vi "Discharge Main.vi"() -> ()   [LabVIEW 2012]
uses:
  Generic Instrument/Data Logger/Data Logger.lvclass
panel:
  out "New set":dbl
  out "Absolute Current set":dbl
  out "Cut-Off Voltage":dbl
  out "Calculated DOD":dbl
  out "Voltage cut off?":bool
  out "Amp hour?":bool
  out "Chroma Load":errorcluster caption="error out" {"code" format="%.0x"}
  out "WT1600":errorcluster
  out "Amp-Hour":dbl
  out "Watt-Hour":dbl
  out "Power":dbl
  out "Current":dbl
  out "Measure":dbl[](array[numeric]) format="%^.4e"
  out "Voltage":dbl
  in  "WT1600":refnum<visa-resource-name>="GPIB0::10::INSTR"
  in  "Chroma 6320 Load":refnum<k15>="GPIB::5::INSTR" caption="resource name"
  out "Time":dbl format="%<%H:%M:%S>t"
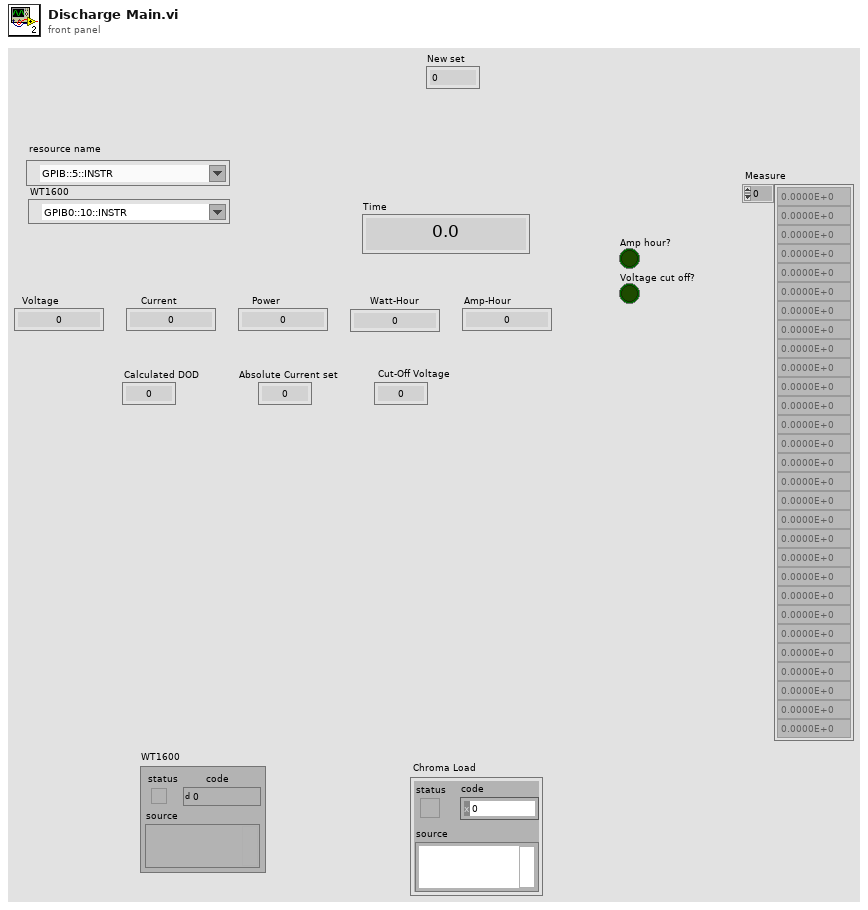
[diagram p1: front panel]
types:
  T1 = cluster{"Amp-Hours":dbl, "% Depth Of Discharge":dbl, "Cut-Off Voltage":dbl}
  T2 = cluster{"Project":string, "Manufactuere":string, "Model":string, "Notes":string}
  T3 = cluster{"V Range (12: 1000)":u16, "A Range (9: 5A)":u16, "A Sensor Ratio(mV/A) (10.0000) ":dbl, "Wiring A (0: 1P2W)":u16}
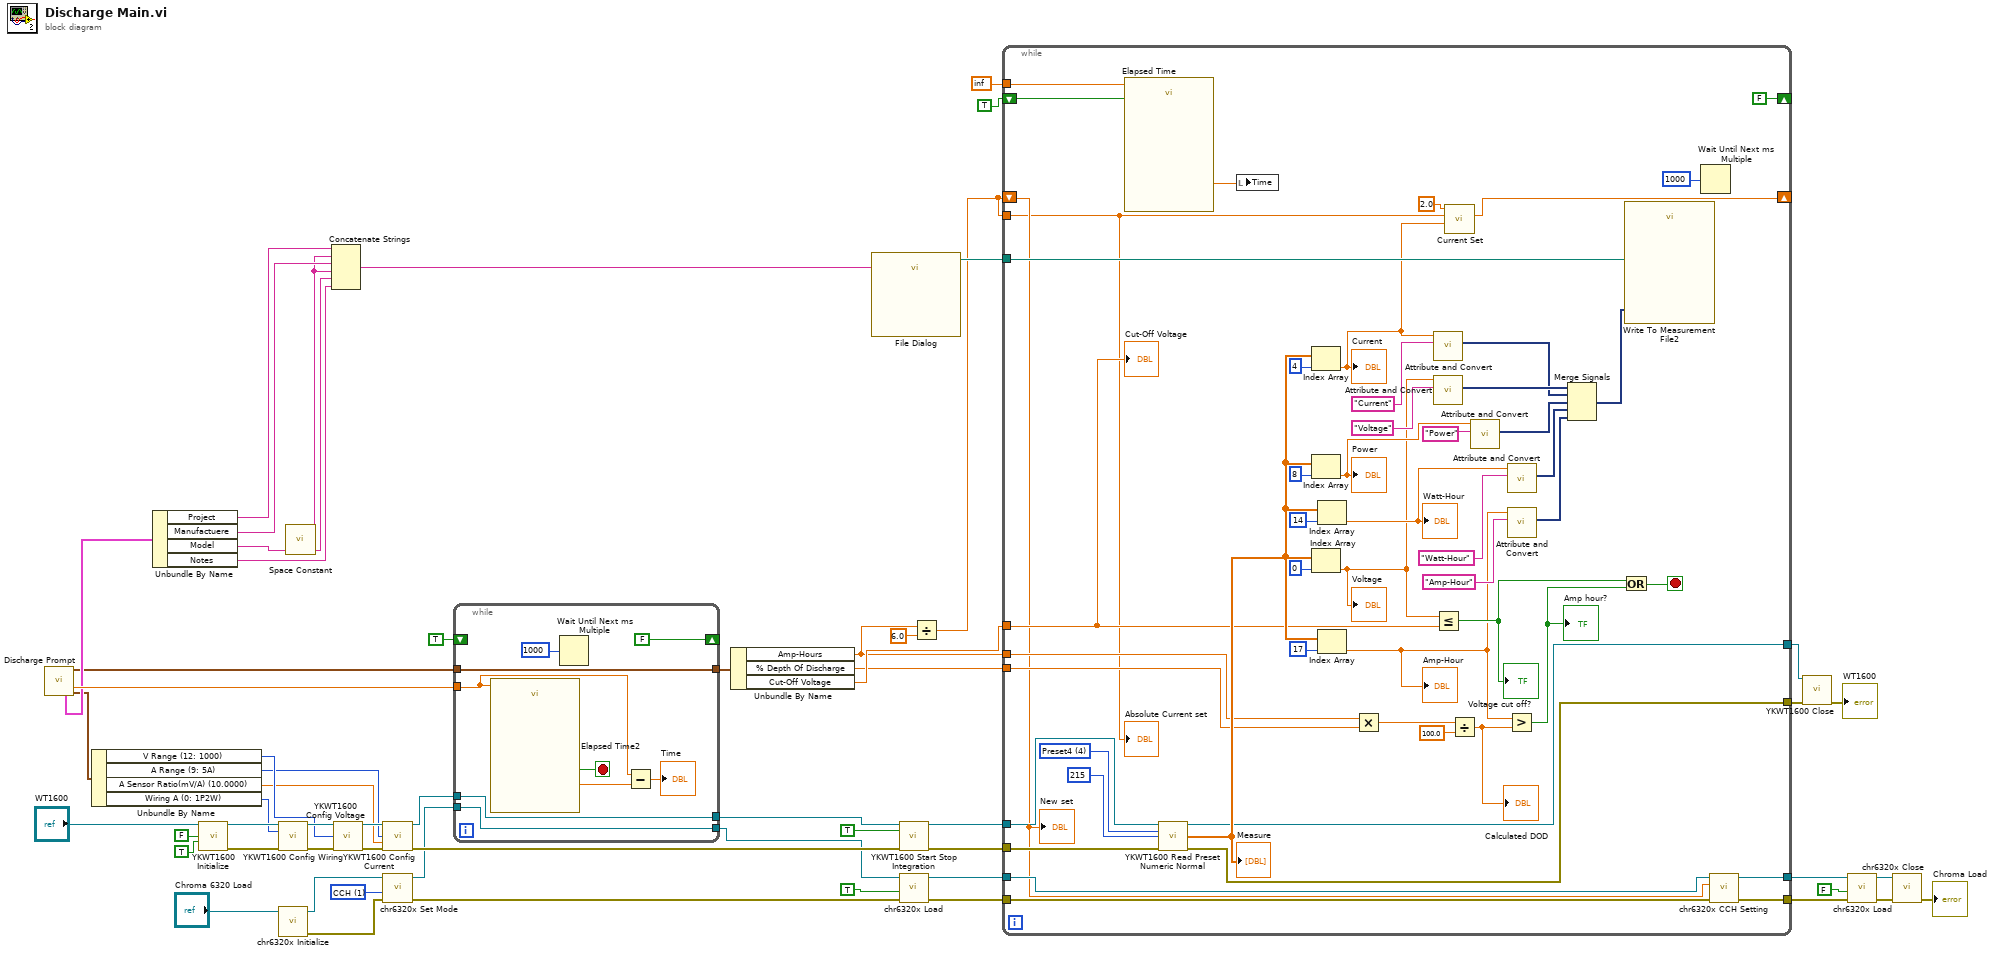
[diagram p0: block diagram]
diagram:
  w53 = 1 items=["CCL", "CCH", "CCDL", "CCDH", "CRL", "CRH", "CVL", "CVH", "CPL", "CPH", "CCEL", "CCEH"] ("Mode (CCL)")
  n1 = call "Discharge Prompt.vi"() -> ("output cluster"=w43:T1, "Warm-Up"=w58:dbl, "Cluster"=w52:T2, "Cluster 2"=w36:T3)  [unwired: 12 in]
  n2 = Unbundle By Name(w36) -> ("V Range (12: 1000)"=w34:u16, "A Range (9: 5A)"=w31:u16, "A Sensor Ratio(mV/A) (10.0000)"=w30:dbl, "Wiring A (0: 1P2W)"=w35:u16)
  n3 = Unbundle By Name(w52) -> ("Project"=w51:string, "Manufactuere"=w50:string, "Model"=w49:string, "Notes"=w47:string)
  n4 = call <instrlib>:"YKWT1600 Initialize.vi"("VISA session (for class)"="WT1600", "ID Query (T: Check)"=FALSE, "Reset (T: Reset)"=TRUE) -> ("VISA session"=w40:refnum<visa-resource-name>, "error out"=w39:errorcluster)  [unwired: 11 in]
  n5 = call <instrlib>:"YKWT1600 Config Wiring.vi"("VISA session"=w40, "Wiring A (0: 1P2W)"=w35, "error in (no error)"=w39) -> ("dup VISA session"=w38:refnum<visa-resource-name>, "error out"=w37:errorcluster)  [unwired: 11 in]
  n6 = call <instrlib>:"chr6320x Initialize.vi"("resource name"="Chroma 6320 Load") -> ("error out"=w54:errorcluster, "instrument handle out"=w55:refnum<k15>)  [unwired: 9 in]
  n7 = call <vilib>:"Space Constant.vi"() -> ("String"=w48:string)
  n8 = Concatenate Strings(w51, w48, w50, w48, w49, w47) -> (w46:string)
  n9 = call <instrlib>:"YKWT1600 Config Voltage.vi"("VISA session"=w38, "V Range (12: 1000)"=w34, "error in (no error)"=w37) -> ("dup VISA session"=w33:refnum<visa-resource-name>, "error out"=w32:errorcluster)  [unwired: 11 in]
  n10 = call <instrlib>:"YKWT1600 Config Current.vi"("VISA session"=w33, "A Range (9: 5A)"=w31, "A Sensor Ratio(mV/A) (10.0000)"=w30, "error in (no error)"=w32) -> ("dup VISA session"=w29:refnum<visa-resource-name>, "error out"=w26:errorcluster)  [unwired: 10 in]
  n11 = call <instrlib>:"chr6320x Set Mode.vi"("error in (no error)"=w54, "Mode (CCL)"=w53, "instrument handle"=w55) -> ("error out"=w19:errorcluster, "instrument handle out"=w20:refnum<k15>)  [unwired: 7 in]
  n12 = while {
    tunnel: w58 -> [w64]
    shift-right: [FALSE] -> _
    shift-left: TRUE -> [_]
    tunnel: [w61] -> w22
    tunnel: w43 -> [w61]
    tunnel: [w60] -> w28
    tunnel: w29 -> [w60]
    tunnel: [w59] -> w17
    tunnel: w20 -> [w59]
    stop <- w66 stop-if-true
    n13 = call "Elapsed Time2"("Time Target (s)"=w64) -> ("Elapsed Time (s)"=w63:dbl, "Time has Elapsed"=w66:bool)  [unwired: 11 in, 6 out]
    n14 = Wait Until Next ms Multiple(millisecond multiple=u32 1000) -> ()  [unwired: 1 out]
    n15 = Subtract(x=w64, y=w63) -> (x-y=→"Time":dbl)
  }
  n16 = Unbundle By Name(w22) -> ("Amp-Hours"=w3:dbl, "% Depth Of Discharge"=w4:dbl, "Cut-Off Voltage"=w21:dbl)
  n17 = call "File Dialog"("default name"=w46) -> ("selected path"=w5:path)  [unwired: 11 in, 3 out]
  n18 = call <instrlib>:"YKWT1600 Start Stop Integration.vi"("VISA session"=w28, "Start/Stop (F: Stop)"=TRUE, "error in (no error)"=w26) -> ("dup VISA session"=w27:refnum<visa-resource-name>, "error out"=w25:errorcluster)  [unwired: 11 in]
  n19 = call <instrlib>:"chr6320x Load.vi"("error in (no error)"=w19, "Load (On)"=TRUE, "instrument handle"=w17) -> ("error out"=w15:errorcluster, "instrument handle out"=w16:refnum<k15>)  [unwired: 7 in]
  n20 = Divide(x=w3, y=6.0) -> (x/y=w1:dbl)
  n21 = while {
    tunnel: w16 -> [w88]
    tunnel: w15 -> [w89]
    shift-right: [FALSE] -> _
    shift-left: TRUE -> [w117]
    tunnel: inf -> [w115]
    tunnel: w27 -> [w113]
    tunnel: w25 -> [w112]
    tunnel: w5 -> [w103]
    tunnel: w3 -> [w83]
    tunnel: w21 -> [w85]
    tunnel: w4 -> [w82]
    tunnel: [w79] -> w14
    tunnel: [w78] -> w13
    tunnel: [w77] -> w9
    tunnel: [w76] -> w8
    shift-right: [w71] -> _
    shift-left: w1 -> [w72]
    tunnel: w1 -> [w69]
    stop <- w87 stop-if-true
    w111 = u16 4 items=["", "Preset1", "Preset2", "Preset3", "Preset4"] ("Preset (2: Preset 2)")
    n22 = call "Elapsed Time"("Time Target (s)"=w115, "Reset"=w117) -> ("Elapsed Time (s)"=w114:dbl)  [unwired: 10 in, 7 out]
    n23 = call <instrlib>:"YKWT1600 Read Preset Numeric Normal.vi"("VISA session"=w113, "Preset (2: Preset 2)"=w111, "Number of Item (15)"=u16 215, "error in (no error)"=w112) -> ("dup VISA session"=w77:refnum<visa-resource-name>, "Measure"=w108:dbl[], "error out"=w76:errorcluster)  [unwired: 8 in, 1 out]
    "Measure" <- w108
    n24 = local write "Time"(w114) -> ()
    n25 = Index Array(array=w108, index=4) -> (element=w68:dbl)
    "Current" <- w68
    n26 = Index Array(array=w108, index=8) -> (element=w100:dbl)
    "Power" <- w100
    n27 = Index Array(array=w108, index=0) -> (element=w86:dbl)
    "Voltage" <- w86
    n28 = Index Array(array=w108, index=14) -> (element=w98:dbl)
    "Watt-Hour" <- w98
    n29 = Index Array(array=w108, index=17) -> (element=w81:dbl)
    "Amp-Hour" <- w81
    n30 = Multiply(x=w83, y=w82) -> (x*y=w75:dbl)
    n31 = call "Attribute and Convert.vi"("Signal Name"="Current", "Number in"=w68) -> ("Dynamic Signal Out"=w94:dynamicdata)  [unwired: 9 in]
    n32 = call "Attribute and Convert.vi"("Signal Name"="Voltage", "Number in"=w86) -> ("Dynamic Signal Out"=w95:dynamicdata)  [unwired: 9 in]
    n33 = Less Or Equal?(x=w86, y=w85) -> (x <= y?=w84:bool)
    "Voltage cut off?" <- w84
    n34 = call "Current Set.vi"("Actual Number"=w68, "Target"=w69, "Percent ceiling"=2.0) -> ("New Set Point"=w71:dbl)  [unwired: 8 in]
    n35 = Divide(x=w75, y=100.0) -> (x/y=w73:dbl)
    "Calculated DOD" <- w73
    n36 = call "Attribute and Convert.vi"("Signal Name"="Power", "Number in"=w100) -> ("Dynamic Signal Out"=w93:dynamicdata)  [unwired: 9 in]
    n37 = call "Attribute and Convert.vi"("Signal Name"="Watt-Hour", "Number in"=w98) -> ("Dynamic Signal Out"=w92:dynamicdata)  [unwired: 9 in]
    n38 = call "Attribute and Convert.vi"("Signal Name"="Amp-Hour", "Number in"=w81) -> ("Dynamic Signal Out"=w91:dynamicdata)  [unwired: 9 in]
    n39 = Greater?(x=w81, y=w73) -> (0:w80:bool)
    "Amp hour?" <- w80
    n40 = Merge Signals(w95, w94, w93, w92, w91) -> (w90:dynamicdata)
    n41 = Or(x=w84, y=w80) -> (x .or. y?=w87:bool)
    n42 = call "Write To Measurement File2"("Signals"=w90, "Filename"=w103) -> ()  [unwired: 15 in, 3 out]
    n43 = Wait Until Next ms Multiple(millisecond multiple=u32 1000) -> ()  [unwired: 1 out]
    n44 = call <instrlib>:"chr6320x CCH Setting.vi"("error in (no error)"=w89, "Current Level (0.0)"=w72, "instrument handle"=w88) -> ("error out"=w78:errorcluster, "instrument handle out"=w79:refnum<k15>)  [unwired: 7 in]
    "Cut-Off Voltage" <- w85
    "Absolute Current set" <- w69
    "New set" <- w72
  }
  n45 = call <instrlib>:"YKWT1600 Close.vi"("VISA session"=w9, "error in (no error)"=w8) -> ("error out"=→"WT1600":errorcluster)  [unwired: 13 in]
  n46 = call <instrlib>:"chr6320x Load.vi"("error in (no error)"=w13, "Load (On)"=FALSE, "instrument handle"=w14) -> ("error out"=w10:errorcluster, "instrument handle out"=w11:refnum<k15>)  [unwired: 7 in]
  n47 = call <instrlib>:"chr6320x Close.vi"("error in (no error)"=w10, "instrument handle"=w11) -> ("error out"=→"Chroma Load":errorcluster)  [unwired: 9 in]
